vi "TDS RF Power Input Read.vi"(6 "Reference Level (dBm)":dbl, 8 "error in (no error)":errorcluster, 9 "Center Frequency (MHz)":dbl, 10 "Signal InstConfig":string, 11 "Address":string) -> (0 "error out":errorcluster, 3 "Power":dbl)   [LabVIEW 2025, in "Interface Functions.lvlib"]
uses:
  Interface Functions.lvlib
  <vilib>/Utility/error.llb/Trim Whitespace One-Sided.vi
  <instrlib>/Agilent U2000 Series/Agilent U2000 Series.lvlib
panel:
  # "RF Power Input Read"
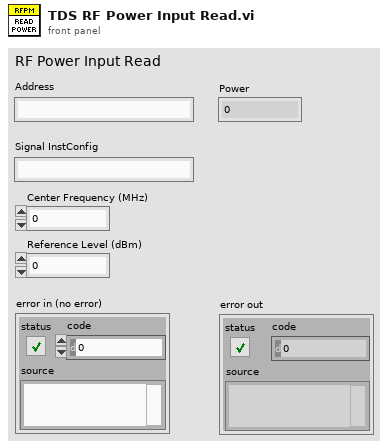
[diagram p1: front panel]
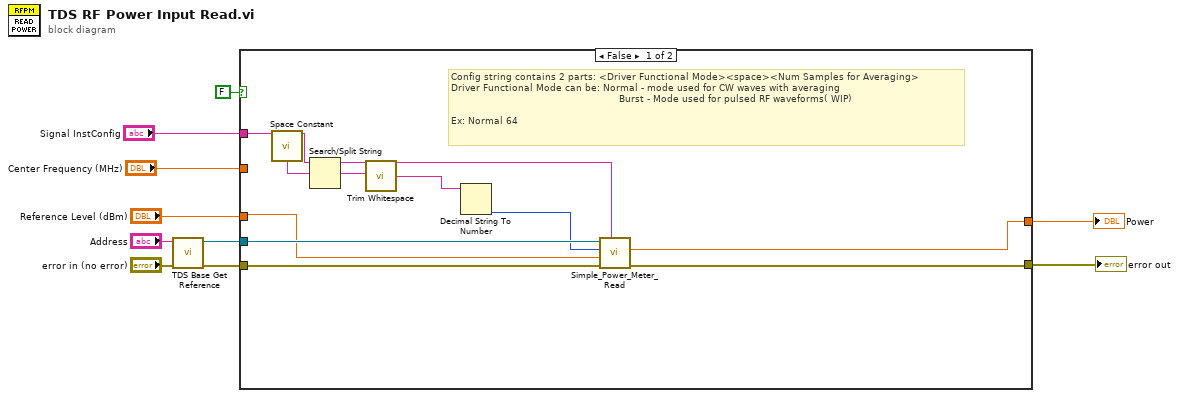
[diagram p0: block diagram]
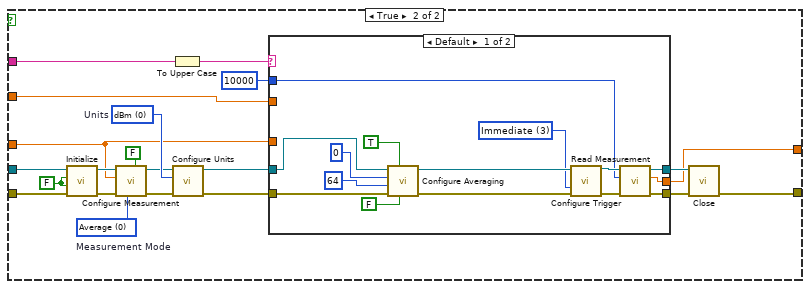
[diagram p2: hidden frame]
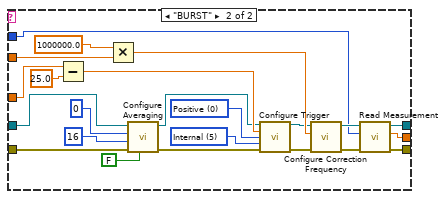
[diagram p3: hidden frame]
diagram:
  n1 = call "TDS Base Get Reference.vi"("error in (no error)"="error in (no error)", "Address"="Address") -> ("error out"=w5:errorcluster, "Reference"=w3:refnum<visa-resource-name>)  [unwired: 8 in]
  n2 = case shown="False" FALSE {
    tunnel: "Signal InstConfig" -> [w19 w42]
    tunnel: [w15 w40] -> w7
    tunnel: [w14 w37] -> w6
    tunnel: w5 -> [w20 w36]
    tunnel: "Center Frequency (MHz)" -> [_ w35]
    tunnel: w3 -> [w21 w34]
    tunnel: "Reference Level (dBm)" -> [w11 w23]
    frame False {
      # "Config string contains 2 parts: <Driver Functional Mode><space><Num Samples for Averaging>\nDriver Functional Mode can be: Normal - mode used for CW waves with averaging\n                                                        Burst - Mode used for pulsed RF waveforms( WIP) \n                                                       \nEx: Normal 64"
      n3 = call <vilib>:"Space Constant.vi"() -> ("String"=w17:string)
      n4 = Search/Split String(string=w19, search string/char (-)=w17) -> (substring before match=w18:string, match + rest of string=w13:string)  [unwired: 1 in, 1 out]
      n5 = call <vilib>:"Trim Whitespace.vi"("string"=w13) -> ("trimmed string"=w12:string)  [unwired: 1 in]
      n6 = Decimal String To Number(string=w12) -> (number=w16:i32)  [unwired: 2 in, 1 out]
      n7 = call "Simple_Power_Meter_Read.vi"("Config String"=w18, "error in (no error)"=w20, "Expected Power(dBm)"=w11, "Sample_count"=w16, "VISA resource name"=w21) -> ("error out"=w15:errorcluster, "Measurement"=w14:dbl)  [unwired: 5 in]
    }
    frame True {
      w29 = 0 items=["Average", "Normal"]  # Measurement Mode
      w30 = u16 0 items=["dBm", "W"]  # Units
      w33 = FALSE ("ID Query (True)")
      n8 = call <instrlib>:"Initialize.vi"("error in (no error)"=w36, "Reset (True)"=w33, "ID Query (True)"=w33, "VISA resource name"=w34) -> ("error out"=w27:errorcluster, "VISA resource name out"=w28:refnum<visa-resource-name>)  [unwired: 6 in]
      n9 = call <instrlib>:"Configure Measurement.vi"("Enable Gate Feed (T: Enable)"=FALSE, "Measurement Function (0: Average)"=w29, "error in (no error)"=w27, "Expected Value (0)"=w23, "VISA resource name"=w28) -> ("error out"=w31:errorcluster, "VISA resource name out"=w26:refnum<visa-resource-name>)  [unwired: 5 in]
      n10 = To Upper Case(1:w42) -> (0:w41:string)
      n11 = call <instrlib>:"Configure Units.vi"("error in (no error)"=w31, "Units (0: dBm)"=w30, "VISA resource name"=w26) -> ("error out"=w25:errorcluster, "VISA resource name out"=w24:refnum<visa-resource-name>)  [unwired: 1 in, 6 out]
      n12 = case shown="Default" w41 {
        tunnel: [w47 w65] -> w39
        tunnel: [w48 w64] -> w38
        tunnel: [w46 w63] -> w37
        tunnel: w25 -> [w44 w62]
        tunnel: w23 -> [_ w61]
        tunnel: w35 -> [_ w60]
        tunnel: w24 -> [w45 w59]
        tunnel: u32 10000 ("Timeout (10000 ms)") -> [w49 w58]
        frame Default {
          w50 = 3 items=["Bus", "External", "Hold", "Immediate", "Internal A", "Internal"] ("Trigger Source (3: Immediate)")
          n13 = call <instrlib>:"Configure Averaging.vi"("Auto Averaging (T: Enable)"=FALSE, "Enable Averaging (T: Enable)"=TRUE, "error in (no error)"=w44, "Averaging Count (4)"=64, "Averaging Buffer Size (1)"=0, "VISA resource name"=w45) -> ("error out"=w54:errorcluster, "VISA resource name out"=w53:refnum<visa-resource-name>)  [unwired: 4 in]
          n14 = call <instrlib>:"Configure Trigger.vi"("VISA resource name"=w53, "Trigger Source (3: Immediate)"=w50, "error in (no error)"=w54) -> ("VISA resource name out"=w52:refnum<visa-resource-name>, "error out"=w51:errorcluster)  [unwired: 11 in]
          n15 = call <instrlib>:"Read Measurement.vi"("error in (no error)"=w51, "Timeout (10000 ms)"=w49, "VISA resource name"=w52) -> ("error out"=w47:errorcluster, "Measurement"=w46:dbl, "VISA resource name out"=w48:refnum<visa-resource-name>)  [unwired: 6 in]
        }
        frame "BURST" {
          w76 = 5 items=["Bus", "External", "Hold", "Immediate", "Internal A", "Internal"] ("Trigger Source (3: Immediate)")
          w77 = u16 0 items=["Positive", "Negative"] ("Trigger Slope (0: Positive)")
          n16 = Subtract(x=w61, y=25.0) -> (x-y=w74:dbl)
          n17 = Multiply(x=1000000.0, y=w60) -> (x*y=w72:dbl)
          n18 = call <instrlib>:"Configure Averaging.vi"("Auto Averaging (T: Enable)"=FALSE, "error in (no error)"=w62, "Averaging Count (4)"=16, "Averaging Buffer Size (1)"=0, "VISA resource name"=w59) -> ("error out"=w67:errorcluster, "VISA resource name out"=w66:refnum<visa-resource-name>)  [unwired: 5 in]
          n19 = call <instrlib>:"Configure Trigger.vi"("VISA resource name"=w66, "Trigger Level (0 dBm)"=w74, "Trigger Slope (0: Positive)"=w77, "Trigger Source (3: Immediate)"=w76, "error in (no error)"=w67) -> ("VISA resource name out"=w70:refnum<visa-resource-name>, "error out"=w71:errorcluster)  [unwired: 9 in]
          n20 = call <instrlib>:"Configure Correction Frequency.vi"("error in (no error)"=w71, "Frequency (5E+7 Hz)"=w72, "VISA resource name"=w70) -> ("error out"=w68:errorcluster, "VISA resource name out"=w69:refnum<visa-resource-name>)  [unwired: 7 in]
          n21 = call <instrlib>:"Read Measurement.vi"("error in (no error)"=w68, "Timeout (10000 ms)"=w58, "VISA resource name"=w69) -> ("error out"=w65:errorcluster, "Measurement"=w63:dbl, "VISA resource name out"=w64:refnum<visa-resource-name>)  [unwired: 6 in]
        }
      }
      n22 = call <instrlib>:"Close.vi"("error in (no error)"=w39, "VISA resource name"=w38) -> ("error out"=w40:errorcluster)  [unwired: 9 in]
    }
  }
  "Power" <- w6
  "error out" <- w7
